vi "wait HOLD.vi"(8 "error in (no error)":errorcluster) -> (0 "error out":errorcluster)   [LabVIEW 2016]
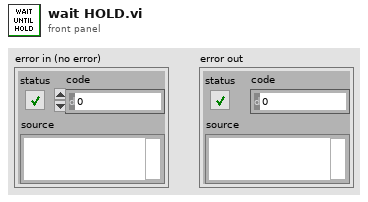
[diagram p1: front panel]
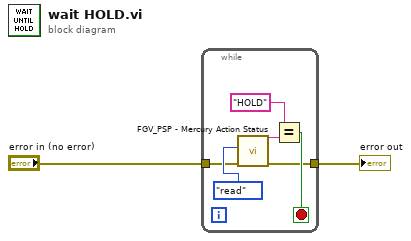
[diagram p0: block diagram]
diagram:
  n1 = while {
    tunnel: "error in (no error)" -> [w4]
    tunnel: [w3] -> w1
    stop <- w6 stop-if-true
    n2 = call "FGV_PSP - Mercury Action Status.vi"("error in"=w4, "Function"=enum16{"write", "read"}."read") -> ("error out"=w3:errorcluster, "Mercury Status 2"=w8:string)  [unwired: 4 in]
    n3 = Equal?(x="HOLD", y=w8) -> (x = y?=w6:bool)
  }
  "error out" <- w1
